vi "Magazine Control 2.0.vi"(0 "Magazine Overflow Power":dbl=1.0, 4 "Magazine Power":dbl=1.0, 6 "Intake Power":dbl=1.0, 8 "Outtake Sensor":bool, 9 "Intake Sensor":bool, 10 "Outtake Button":bool, 11 "Intake Button":bool) -> (2 "Magazine":dbl, 3 "Intake":dbl)   [LabVIEW 2019]
uses:
  Magazine State.ctl
panel:
  out "Current State":T1
  in  "Initial State":T1
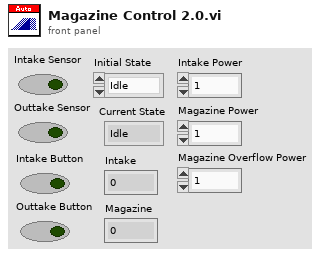
[diagram p1: front panel]
types:
  T1 = typedef "Magazine State.ctl" = enum16{"Idle", "Intake Idle", "Move Cell", "Prevent Overflow", "Outtake Idle", "Shoot"}
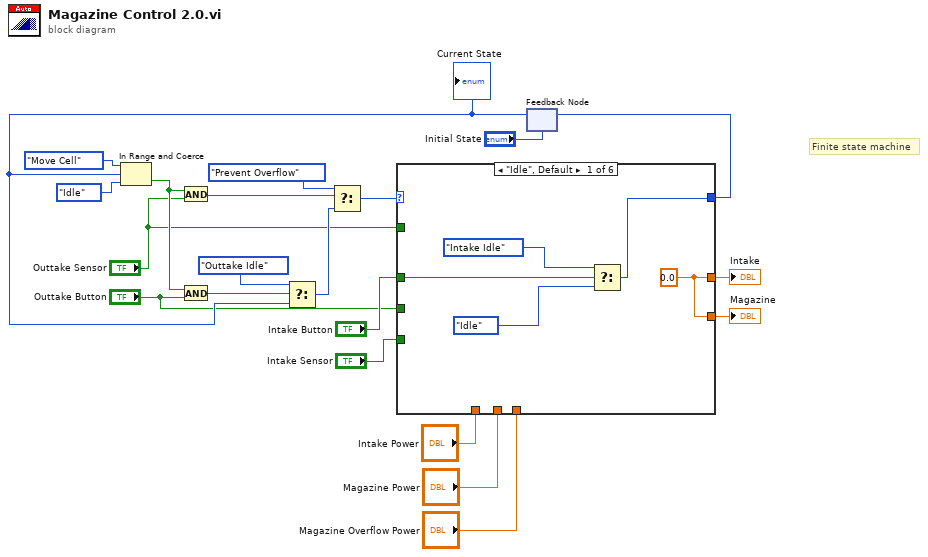
[diagram p0: block diagram]
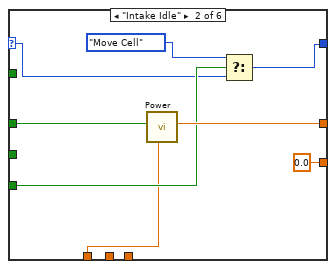
[diagram p2: hidden frame]
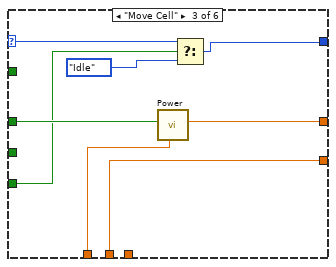
[diagram p3: hidden frame]
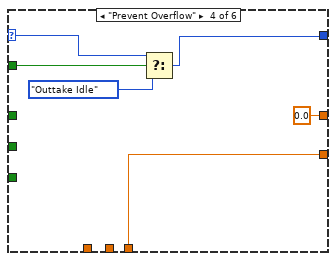
[diagram p4: hidden frame]
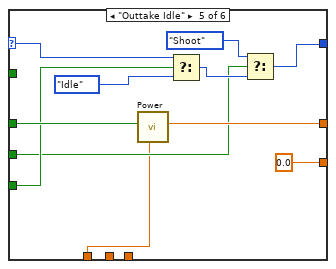
[diagram p5: hidden frame]
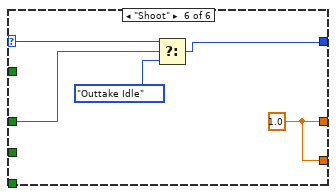
[diagram p6: hidden frame]
diagram:
  # "Finite state machine"
  n1 = feedback #1("Initial State") -> (w10:T1)
  "Current State" <- w10
  n2 = In Range and Coerce(upper limit=Magazine_State."Move Cell" ("lower limit"), x=w10, lower limit=Magazine_State."Idle") -> (In Range?=w14:bool)  [unwired: 1 out]
  n3 = And(x=w14, y="Outtake Sensor") -> (x .and. y?=w15:bool)
  n4 = And(x=w14, y="Outtake Button") -> (x .and. y?=w13:bool)
  n5 = Select(t=Magazine_State."Outtake Idle" ("lower limit"), s=w13, f=w10) -> (s? t:f=w12:T1)
  n6 = Select(t=Magazine_State."Prevent Overflow" ("lower limit"), s=w15, f=w12) -> (s? t:f=w17:T1)
  n7 = case shown="\"Idle\", Default" w17 {
    selector: w17 -> [_ w28 w39 w45 w55 w63]
    tunnel: "Intake Button" -> [w25 w34 w42 _ w59 w64]
    tunnel: [w23 w33 w36 0.0 ("Output") w58 w60] -> w9
    tunnel: [w23 0.0 w41 w48 0.0 ("Magazine Overflow Power") w60] -> w8
    tunnel: "Intake Power" -> [_ w27 w35 _ w49 _]
    tunnel: "Intake Sensor" -> [_ w31 w40 _ w56 _]
    tunnel: "Magazine Power" -> [_ _ w41 _ _ _]
    tunnel: [w22 w30 w37 w44 w50 w61] -> w4
    tunnel: "Magazine Overflow Power" -> [_ _ _ w48 _ _]
    tunnel: "Outtake Sensor" -> [_ _ _ w46 _ _]
    tunnel: "Outtake Button" -> [_ _ _ _ w52 _]
    frame "Idle", Default {
      w23 = 0.0
      n8 = Select(t=Magazine_State."Intake Idle", s=w25, f=Magazine_State."Idle") -> (s? t:f=w22:T1)
    }
    frame "Intake Idle" {
      n9 = call "Power.vi"("Positive Power"=w27, "Positive"=w34) -> ("Output"=w33:dbl)  [unwired: 9 in]
      n10 = Select(t=Magazine_State."Move Cell" ("lower limit"), s=w31, f=w28) -> (s? t:f=w30:T1)
    }
    frame "Move Cell" {
      n11 = call "Power.vi"("Positive Power"=w35, "Positive"=w42) -> ("Output"=w36:dbl)  [unwired: 9 in]
      n12 = Select(t=w39, s=w40, f=Magazine_State."Idle") -> (s? t:f=w37:T1)
    }
    frame "Prevent Overflow" {
      n13 = Select(t=w45, s=w46, f=Magazine_State."Outtake Idle" ("lower limit")) -> (s? t:f=w44:T1)
    }
    frame "Outtake Idle" {
      n14 = call "Power.vi"("Positive Power"=w49, "Positive"=w59) -> ("Output"=w58:dbl)  [unwired: 9 in]
      n15 = Select(t=w55, s=w56, f=Magazine_State."Idle") -> (s? t:f=w53:T1)
      n16 = Select(t=Magazine_State."Shoot" ("f"), s=w52, f=w53) -> (s? t:f=w50:T1)
    }
    frame "Shoot" {
      w60 = 1.0 ("Magazine Overflow Power")
      n17 = Select(t=w63, s=w64, f=Magazine_State."Outtake Idle") -> (s? t:f=w61:T1)
    }
  }
  "Intake" <- w9
  "Magazine" <- w8
  n18 = feedback-in #1(w4) -> ()
